vi "Read Allow.vi"(8 "error in (no error)":errorcluster, 9 "Interlock in (False)":bool, 11 "Interlock Chain in":refnum<class "Interlock Chain.lvclass">) -> (0 "error out":errorcluster, 1 "Interlock out":bool, 2 "Allow":refnum<class "Interlock.lvclass">[](array[class]), 3 "Interlock Chain out":refnum<class "Interlock Chain.lvclass">)   [LabVIEW 2015, in "Interlocks.lvlib" / "Interlock Chain.lvclass"]
uses:
  Interlock Chain.lvclass
  Interlock/Interlock.lvclass
  Interlock Chain.lvclass/Interlock Chain.ctl
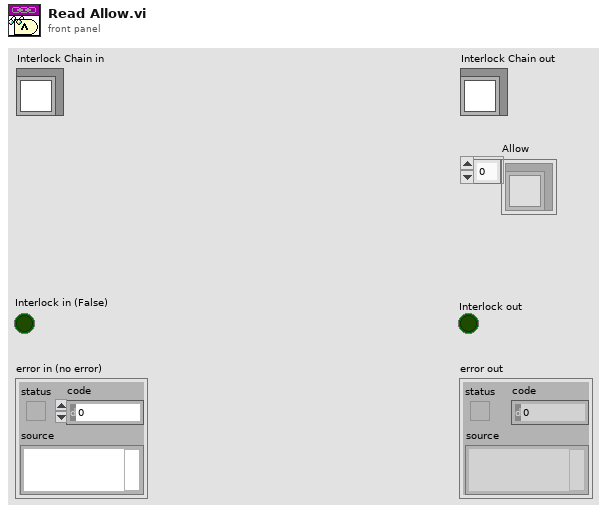
[diagram p1: front panel]
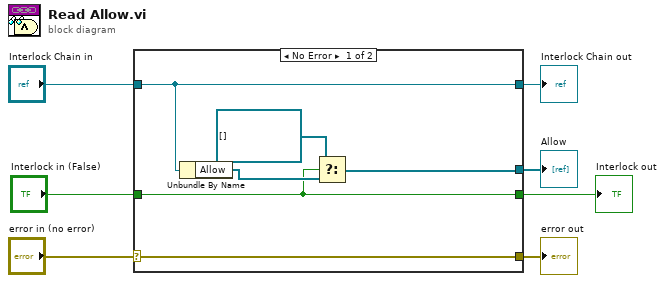
[diagram p0: block diagram]
diagram:
  n1 = case shown="No Error" "error in (no error)" {
    selector: "error in (no error)" -> [w13 w14]
    tunnel: [w13 w14] -> w6
    tunnel: [w12 w15] -> w4
    tunnel: "Interlock Chain in" -> [w12 w15]
    tunnel: [w11 _] -> w3
    tunnel: "Interlock in (False)" -> [w8 _]
    tunnel: [w8 _] -> w1
    frame No Error {
      n2 = Unbundle By Name(w12) -> ("Allow"=w10:refnum<class "Interlock.lvclass">[])
      n3 = Select(t=refnum<class "Interlock.lvclass">[] [], s=w8, f=w10) -> (s? t:f=w11:refnum<class "Interlock.lvclass">[])
    }
    frame Error {
    }
  }
  "error out" <- w6
  "Interlock Chain out" <- w4
  "Allow" <- w3
  "Interlock out" <- w1
